vi "Sweep_AIWFM_time.vi"(8 "error in (no error)":errorcluster, 11 "Transport":refnum<class "Transport.lvclass">) -> (0 "error out":errorcluster, 3 "Transport.lvclass":refnum<class "Transport.lvclass">)   [LabVIEW 2019, in "Transport.lvclass"]
uses:
  Transport.lvclass
  <userlib>/LevyLab/Instrument Framework/Instrument Types/Cryostat/Instrument.Cryostat.lvclass
  Control Experiment/Control Experiment.lvclass
  Control Experiment/Typedefs/Instrument Classes--cluster.ctl
  <userlib>/LevyLab/Instrument Framework/Instrument Types/VSource/Instrument.VSource.lvclass
  <userlib>/LevyLab/Instrument Framework/Instrument Types/VNA/Instrument.VNA.lvclass
  <userlib>/LevyLab/Instrument Framework/Instrument Types/Strain/Instrument.Strain.lvclass
  <userlib>/LevyLab/Instrument Framework/Instrument Types/CBridge/Instrument.CBridge.lvclass
  <vilib>/Waveform/WDTOps.llb/WDT Append Waveforms DBL.vi
  <vilib>/PRIrvin/XY Utilities/xy_utilities.lvlib
  <vilib>/PRIrvin/XY Utilities/subVIs/Waveform to XY (single).vi
  <vilib>/PRIrvin/XY Utilities/subVIs/Get X and Y (single).vi
  <userlib>/LevyLab/Lockin-Multichannel/Instrument.DAQ/Typedefs/Sweep.Configuration--Cluster.ctl
  <userlib>/LevyLab/Lockin-Multichannel/Instrument.DAQ/Instrument.DAQ.lvclass
  <userlib>/LevyLab/Lockin-Multichannel/Instrument.DAQ/Typedefs/Sweep.Channel--Cluster.ctl
  <userlib>/LevyLab/Instrument Framework/Instrument Types/Delay Line/Instrument.DelayLine.lvclass
  <userlib>/LevyLab/Lockin-Multichannel/Instrument.DAQ/Typedefs/Sweep.Channel--Cluster--Array.ctl
  <userlib>/LevyLab/Instrument Framework/Instrument Types/Lockin/Instrument.LockinAPI.lvclass
  <userlib>/LevyLab/Instrument Framework/Instrument Types/Amplifier/Instrument.Amplifier.lvclass
  <userlib>/LevyLab/Lockin-Multichannel/Instrument.DAQ/Typedefs/Sweep.Pattern--Enum.ctl
  <userlib>/LevyLab/Lockin-Multichannel/Instrument.Lockin/Instrument.Lockin.lvclass
  <userlib>/LevyLab/Lockin-Multichannel/Instrument.DAQ/Typedefs/Get State-enum.ctl
panel:
  out "elapsed time (s)":u32=36594
  out "time b/w points (ms)":u32=533
  in  "Stop":bool
  in  "Tab Control":enum32{"Control", "Waveform", "Other"}(tab)
  in  "Sweep Time (s)":dbl=10.0 format="%#_3p"
  in  "Initial Wait (s)":u32=1
  in  "Return to Start":bool=TRUE
  in  "wait (ms)":u32=500
  in  "Experiment Description":string="SA40321H:\nT=80mK, BG=0V, B=-9T\nLoop 0: sgR: -1V to 1V, 20mV step\nInner loop: I+/I-: 28/2   -180mV to 220mV, sweep time 10s\nsgL (lead 1): 0V\nsgR (lead 3): sweep\n    \nI+/I-: 28/2   -180mV to 220mV, sweep time 10s\nV+/V-: 5/2\nsgL-lead 1; sgR-lead 3\n\ntc: 100ms\norder: 4\n\n"
  in  "Experiment Folder":string="01-sgR IV for RD"
  in  "Channels":T1[](array[typedef]) {"Table" format="%#_1f"; "Channel" min=1 max=128; "Start" format="%#_6p"; "End" format="%#_6p"}
  out "AO":waveform(dbl)(graph)={"t0"=timestamp(3666661573.979815 s since 1904-01-01), "dt"=0.0009999999996825864, "Y"=[]}
  out "AI vs AO":cluster{"Y":dbl[], "Y":dbl[]}[](graph)
  out "AI":waveform(dbl)[](graph)
  out "Status":T3=enum."created"
  out "Current State":string="File: Save"
  # "*** These controls are only read if this VI is the top level. If is is called from Sweep Control then the folder and comments come from Sweep Control.vi ***"
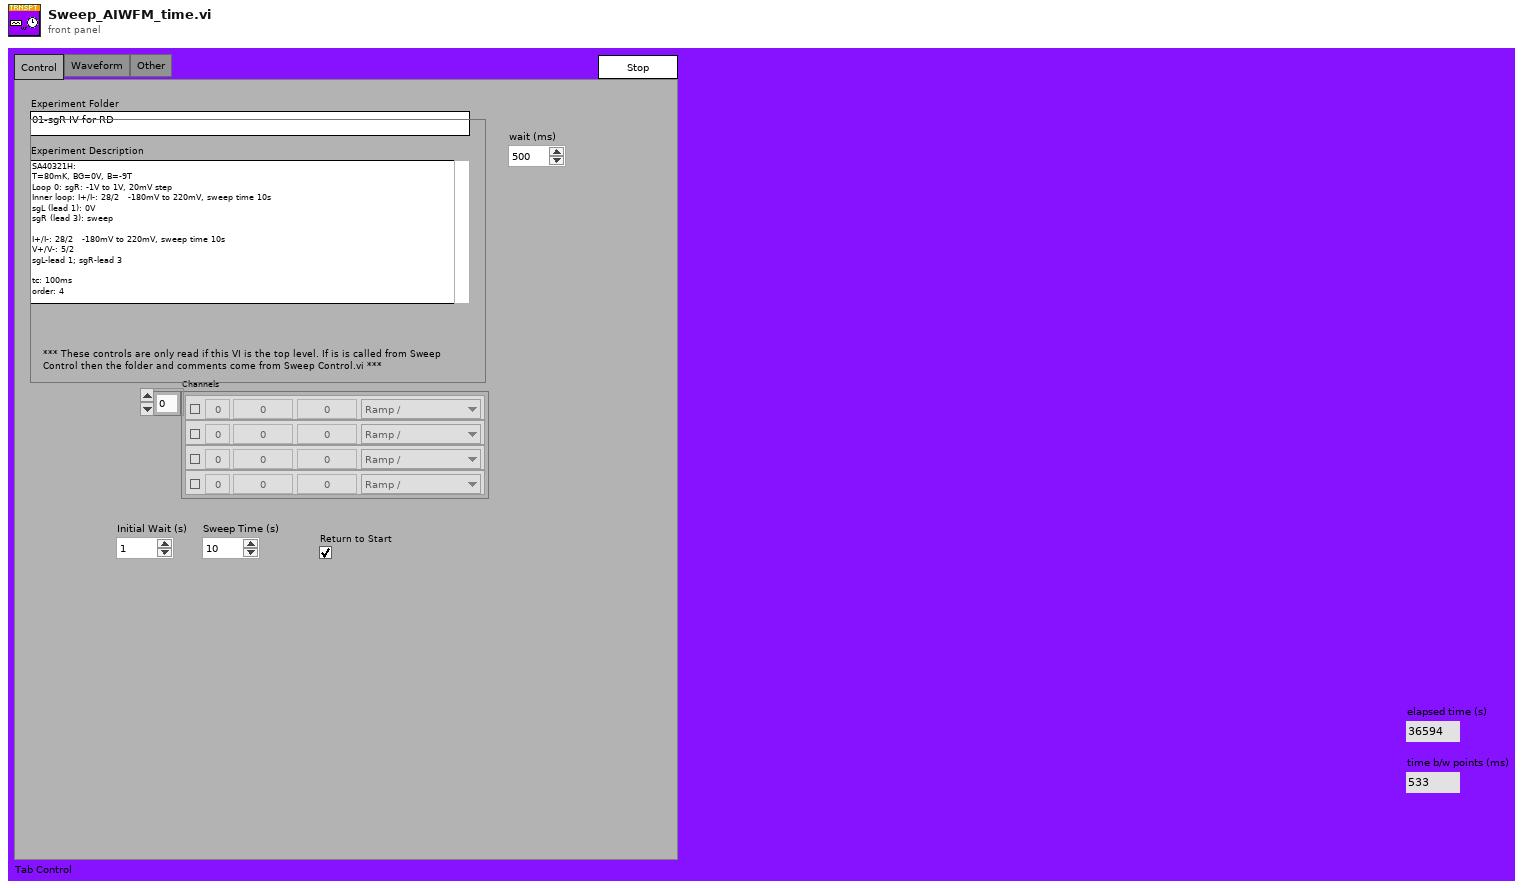
[diagram p1: front panel]
types:
  T1 = typedef "Instrument.Lockin.lvlib/Instrument.DAQ.lvclass/Sweep.Channel--Cluster.ctl" = cluster{"Enable?":bool, "Channel":u16, "Start":dbl, "End":dbl, "Pattern":T2, "Table":dbl[]}
  T2 = typedef "Instrument.Lockin.lvlib/Instrument.DAQ.lvclass/Sweep.Pattern--Enum.ctl" = enum16{"Ramp /", "Ramp /\\", "Smooth Ramp _/", "Smooth Ramp _/\\_", "Table"}
  T3 = typedef "Instrument.Lockin.lvlib/Instrument.DAQ.lvclass/Get State-enum.ctl" = enum16{"idle", "created", "started", "stopped", "sweeping"}
  T4 = enum32{"Invalid", "Standard", "Closed", "Hidden", "Minimized", "Maximized"}
  T5 = enum32{"invalid app kind", "Development System", "Run Time System", "Student Edition", "Embedded LabVIEW", "Evaluation", "Custom"}
  T6 = typedef "Control Experiment.lvclass/Instrument Classes--cluster.ctl" = cluster{"DAQ":refnum<class "Instrument.LockinAPI.lvclass">, "Amplifier":refnum<class "Instrument.Amplifier.lvclass">, "Temperature":refnum<class "Instrument.Cryostat.lvclass">, "Magnet":refnum<class "Instrument.Cryostat.lvclass">, "Rotator":refnum<class "Instrument.Cryostat.lvclass">, "Level":refnum<class "Instrument.Cryostat.lvclass">, "Capacitance":refnum<class "Instrument.CBridge.lvclass">, "Delay Line":refnum<class "Instrument.DelayLine.lvclass">, "Strain Cell":refnum<class "Instrument.Strain.lvclass">, "VNA":refnum<class "Instrument.VNA.lvclass">, "Source":refnum<class "Instrument.VSource.lvclass">}
  T7 = typedef "Instrument.Lockin.lvlib/Instrument.DAQ.lvclass/Sweep.Configuration--Cluster.ctl" = cluster{"Sweep Time (s)":dbl, "Initial Wait (s)":dbl, "Return to Start":bool, "Channels":T8}
  T8 = typedef "Instrument.Lockin.lvlib/Instrument.DAQ.lvclass/Sweep.Channel--Cluster--Array.ctl" = T1[]
  T9 = cluster{"Core":cluster{"Current VI Reference":refnum<vi>, "Close Panel on Exit?":bool}, "Transport":refnum<class "Transport.lvclass">, "C.E.":refnum<class "Control Experiment.lvclass">, "Notifier":refnum<notifier>, "Instruments":T6, "path":path, "time":dbl, "temperature":dbl, "magnet field":dbl, "AI XY (new)":cluster{dbl[], dbl[]}[], "AI XY (all)":cluster{dbl[], dbl[]}[], "AI Waveform (s)":waveform(dbl)[], "t0":timestamp, "ms [0]":u32, "ms [i]":u32, "AO Waveform (s)":waveform(dbl)[], "Execution:State":enum32{"Bad", "Idle", "Run top level", "Running"}}
  T10 = enum32{"Bad", "Idle", "Run top level", "Running"}
  T11 = cluster{"Current VI Reference":refnum<vi>, "Close Panel on Exit?":bool}
  T12 = typedef "Instrument.LockinAPI.lvclass/LockinAPI.getState.states--enum.ctl" = enum16{"idle", "created", "started", "stopped", "sweeping"}
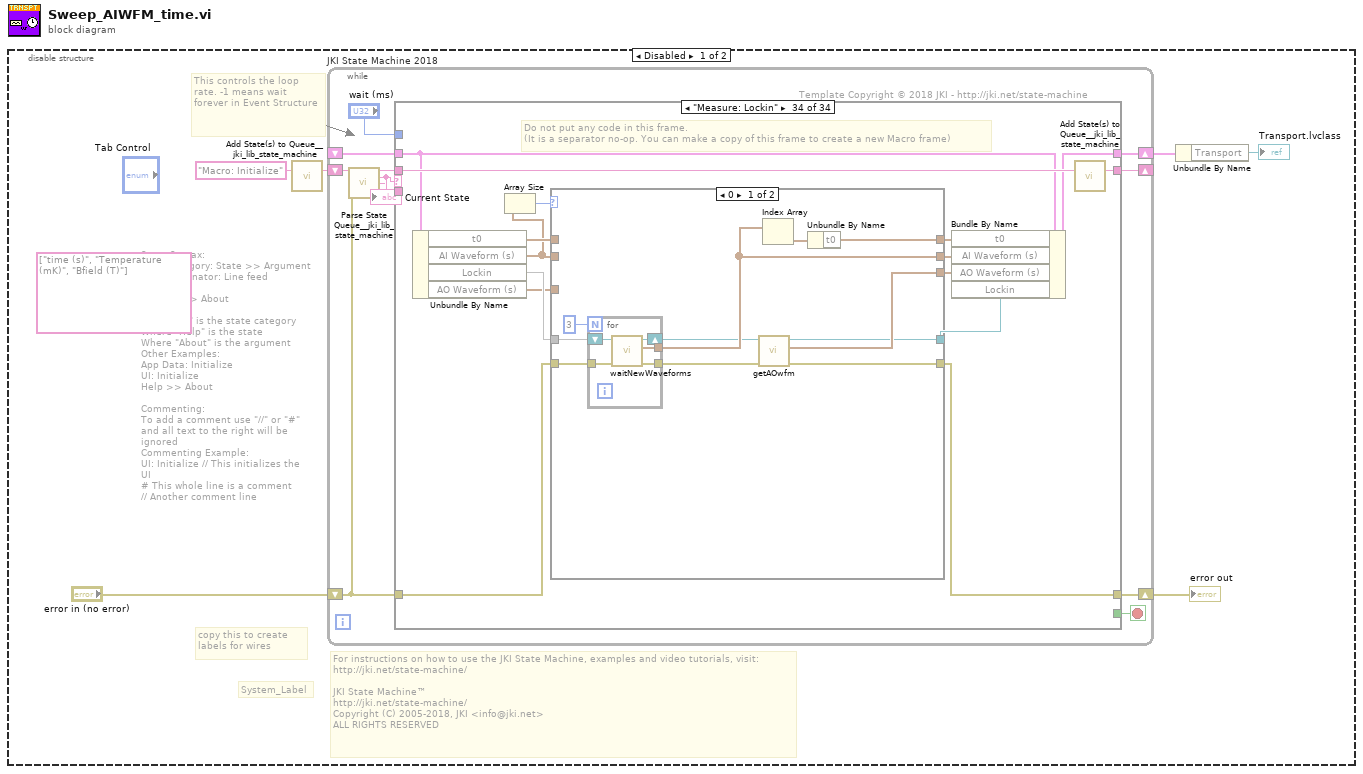
[diagram p0: block diagram]
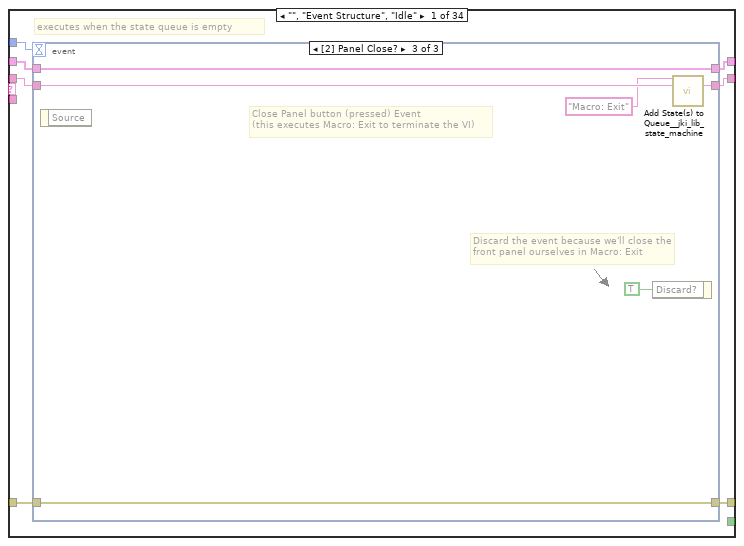
[diagram p2: hidden frame]
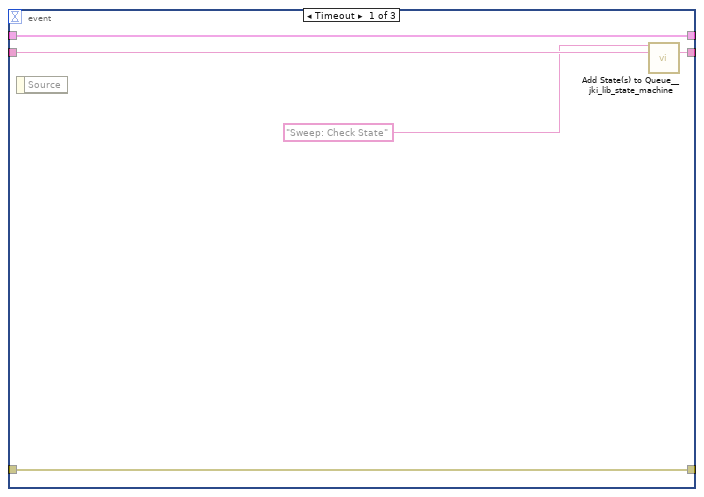
[diagram p3: hidden frame]
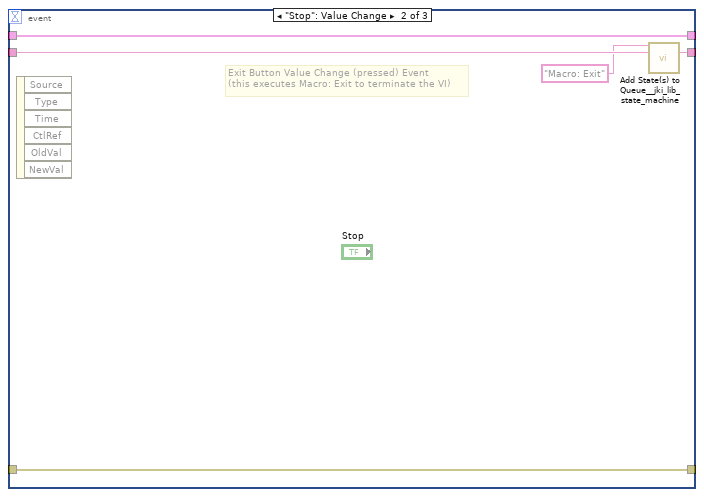
[diagram p4: hidden frame]
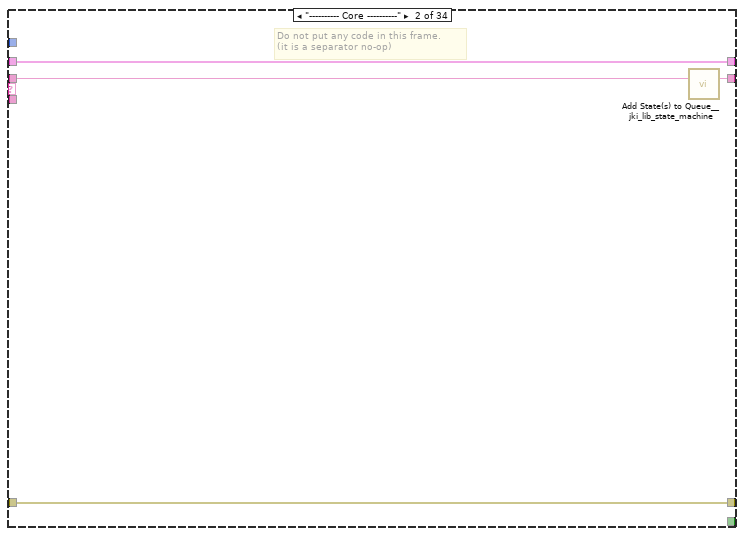
[diagram p5: hidden frame]
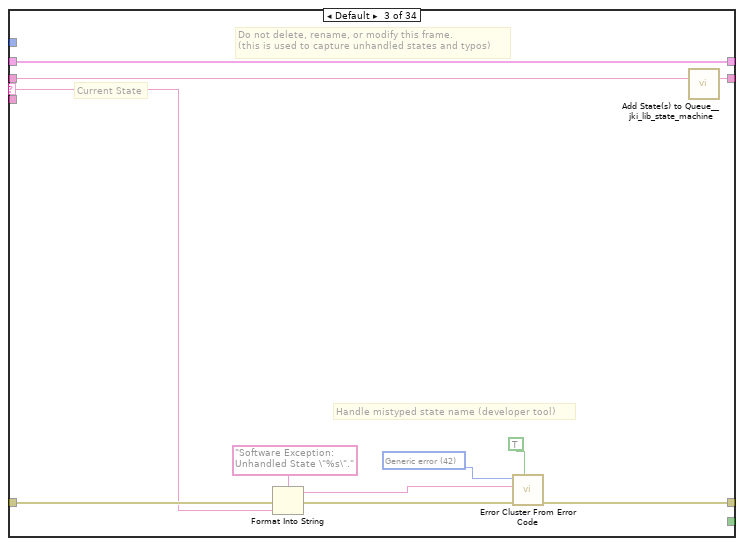
[diagram p6: hidden frame]
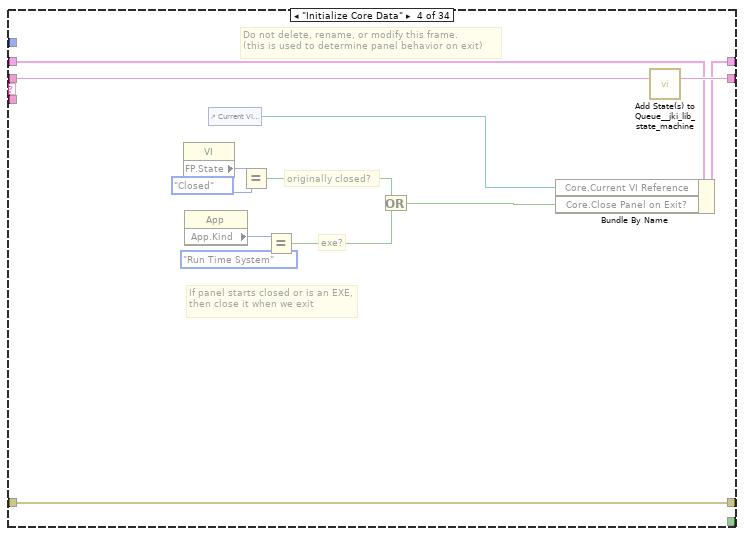
[diagram p7: hidden frame]
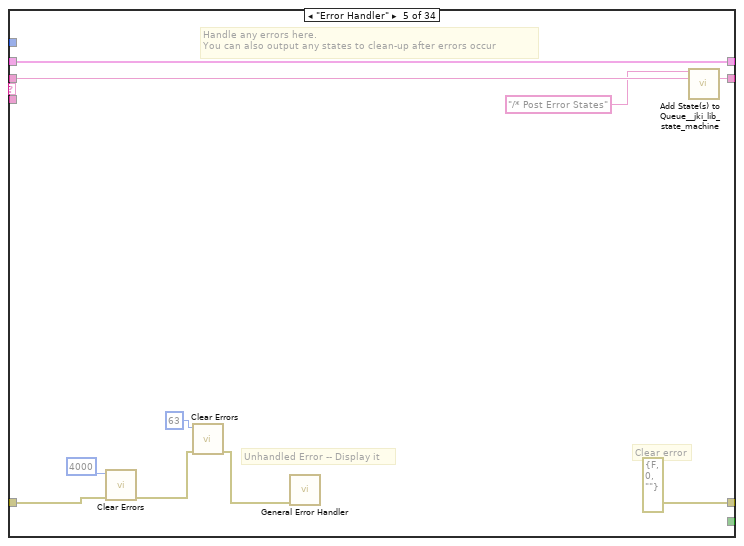
[diagram p8: hidden frame]
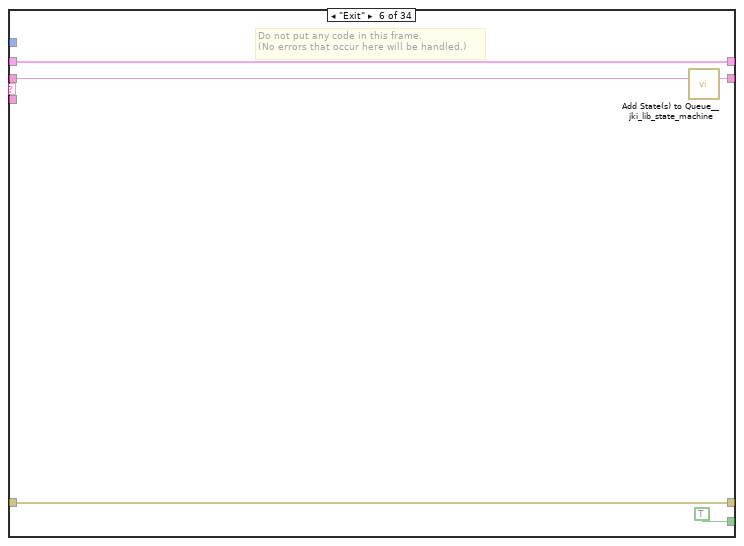
[diagram p9: hidden frame]
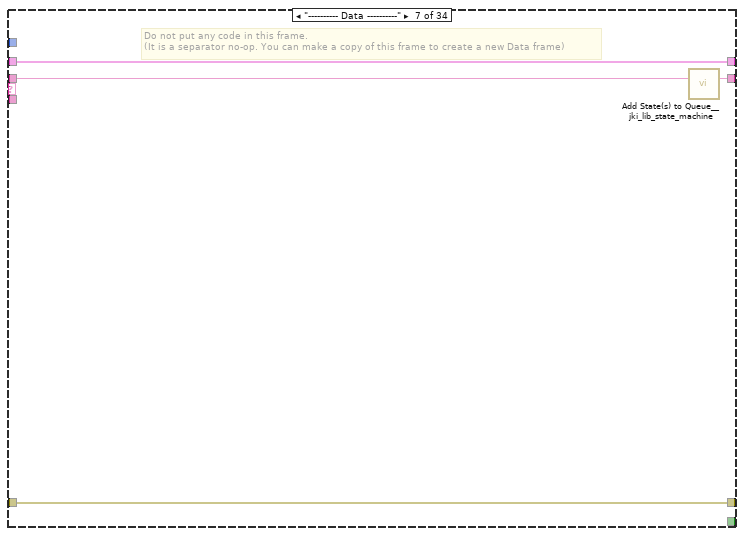
[diagram p10: hidden frame]
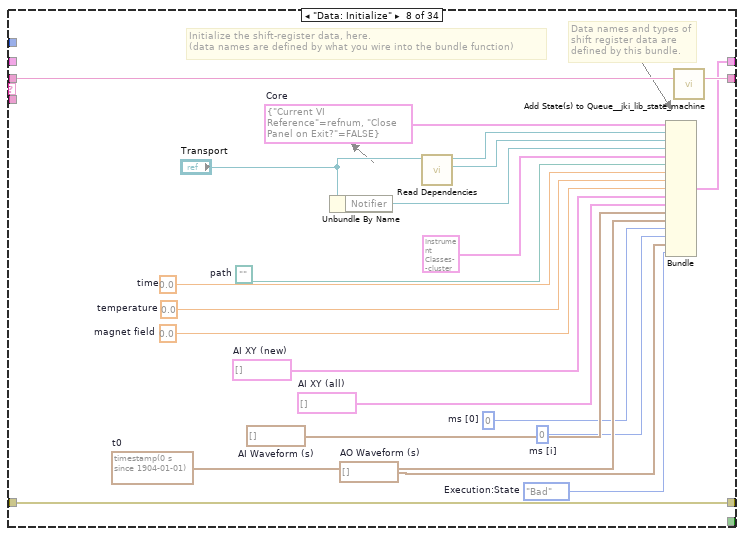
[diagram p11: hidden frame]
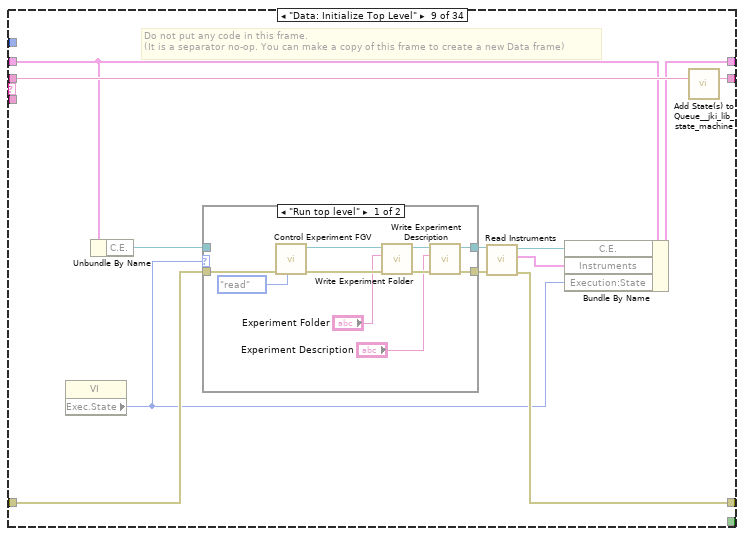
[diagram p12: hidden frame]
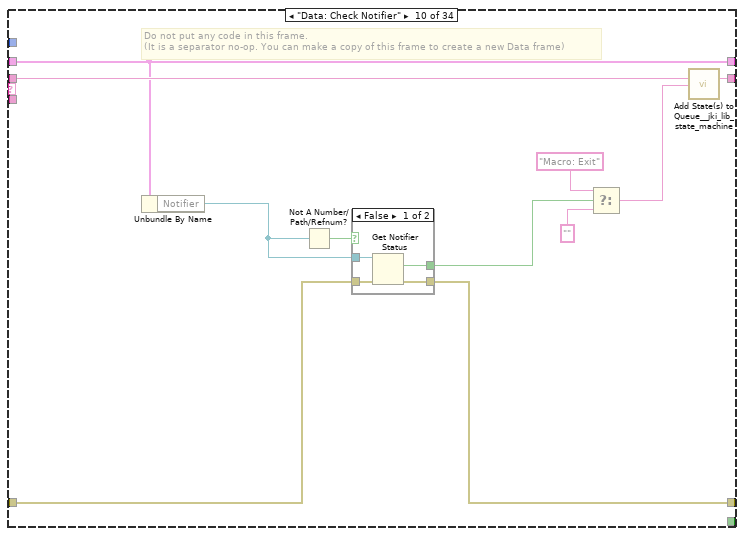
[diagram p14: hidden frame]
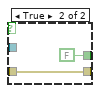
[diagram p15: hidden frame]
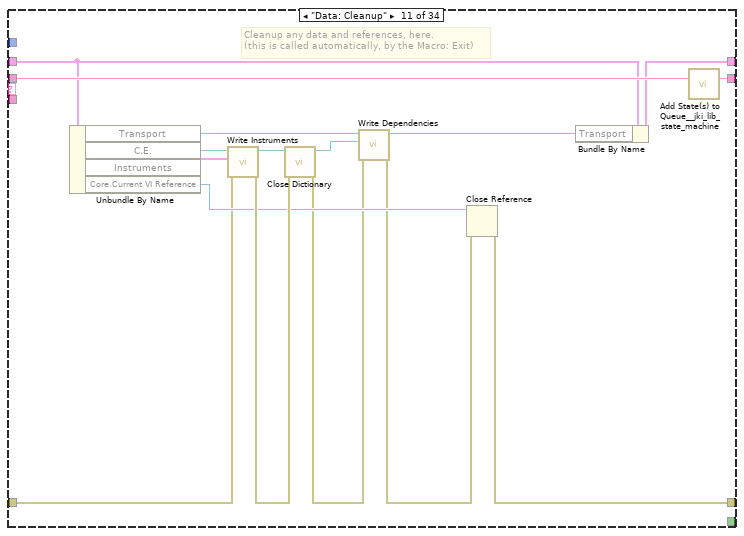
[diagram p16: hidden frame]
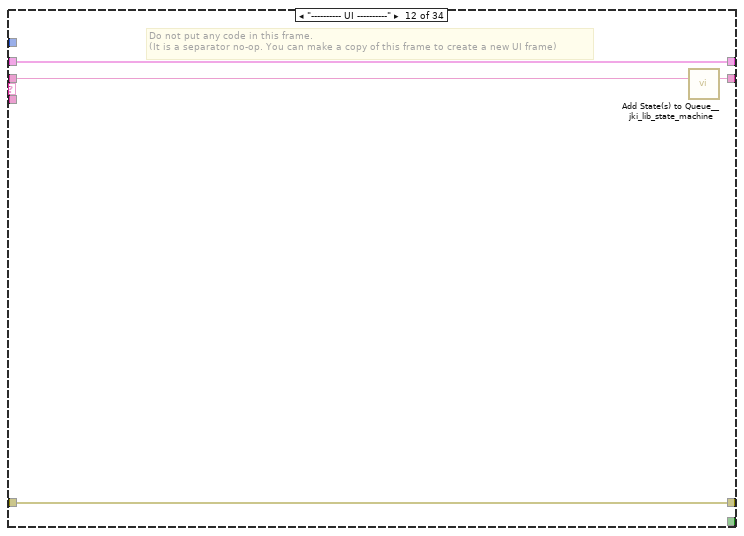
[diagram p17: hidden frame]
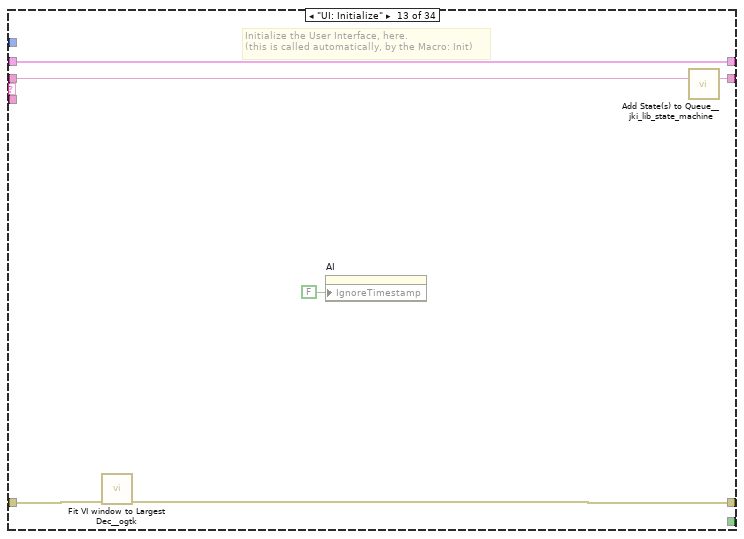
[diagram p18: hidden frame]
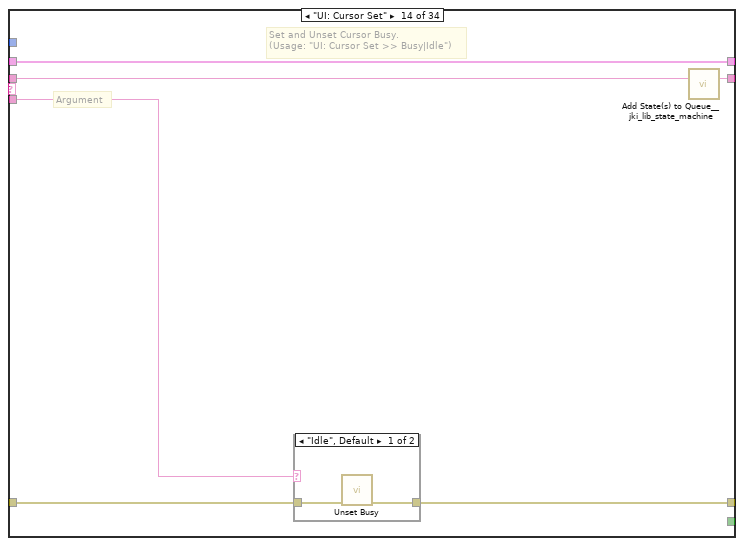
[diagram p19: hidden frame]
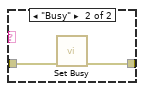
[diagram p20: hidden frame]
diagram:
  n1 = disable-structure shown="Disabled" {
    frame Disabled {
      (unwired) string[] ["time (s)", "Temperature (mK)", "Bfield (T)"] ("wavenames (.Vx, etc)")
      # "For instructions on how to use the JKI State Machine, examples and video tutorials, visit:\nhttp://jki.net/state-machine/\n\nJKI State Machine™\nhttp://jki.net/state-machine/\nCopyright (C) 2005-2018, JKI <info@jki.net>\nALL RIGHTS RESERVED"
      # "State Syntax:\nStateCategory: State >> Argument\nLine Terminator: Line feed\nExample:\nUI: Help >> About\n\nWhere \"UI\" is the state category\nWhere \"Help\" is the state\nWhere \"About\" is the argument\nOther Examples:\nApp Data: Initialize\nUI: Initialize\nHelp >> About\n\nCommenting:\nTo add a comment use \"//\" or \"#\" and all text to the right will be ignored\nCommenting Example:\nUI: Initialize // This initializes the UI\n# This whole line is a comment\n// Another comment line"
      # "copy this to create labels for wires"
      # "This controls the loop rate. -1 means wait forever in Event Structure"
      # "System_Label"
      n2 = call <vilib>:"Add State(s) to Queue__jki_lib_state_machine.vi"("State(s) in (\"\")"="Macro: Initialize") -> ("States Out"=w6:string)  [unwired: 14 in]
      n3 = while "JKI State Machine 2018" {
        shift-right: [w10] -> w2
        shift-left: _ -> [w9]
        shift-right: [w13] -> w3
        shift-left: "error in (no error)" -> [w8]
        shift-right: [w12] -> _
        shift-left: w6 -> [w14]
        stop <- w11 stop-if-true
        # "Template Copyright © 2018 JKI - http://jki.net/state-machine"
        n4 = call <vilib>:"Parse State Queue__jki_lib_state_machine.vi"("State Queue"=w14, "Error In (no error)"=w8) -> ("Remaining States"=w16:string, "Current State"=w17:string, "Arguments"=w15:string)  [unwired: 11 in]
        "Current State" <- w17
        n5 = case shown="\"Measure: Lockin\"" w17 {
          selector: w17 -> [_ _ w45 _ _ _ _ _ _ _ _ _ _ _ _ _ _ _ _ _ _ _ _ _ _ _ _ _ _ _ _ _ _ _]
          tunnel: w16 -> [w24 w44 w49 w68 w78 w83 w87 w109 w121 w144 w166 w170 w176 w182 w193 w270 w288 w292 w297 w302 w310 w320 w324 w347 w371 w387 w397 w405 w415 w421 w432 w445 w458 w473]
          tunnel: w15 -> [_ _ _ _ _ _ _ _ _ _ _ _ _ w177 w187 _ _ _ _ _ _ _ _ _ _ _ _ _ _ _ _ _ _ _]
          tunnel: w9 -> [w22 w41 w47 w61 w75 w81 w84 _ w117 w141 w153 w167 w174 w180 w189 w268 w276 w289 w294 w299 w307 w317 w321 w345 w368 w376 w390 w398 w406 w418 w428 w441 w456 w470]
          tunnel: [w21 w42 w51 w65 errorcluster {"status"=FALSE, "code"=0, "source"=""} ("error out") w80 w85 w106 w111 w140 w151 w168 w172 w178 w190 w267 w278 w290 w295 w300 w308 w318 w322 w344 w369 w384 w388 w401 w410 w419 w422 w434 w451 w464] -> w13
          tunnel: w8 -> [w20 w42 w50 w65 w72 w80 w85 w106 w116 w139 w152 w168 w173 w179 w191 w267 w279 w290 w295 w300 w308 w318 w322 w340 w369 w385 w394 w402 w411 w419 w425 w442 w450 w465]
          tunnel: [w23 w43 w48 w67 w77 w82 w86 w108 w120 w143 w165 w169 w175 w181 w192 w269 w287 w291 w296 w301 w309 w319 w323 w346 w370 w386 w396 w404 w414 w420 w431 w444 w457 w472] -> w12
          tunnel: [_ _ _ _ _ TRUE _ _ _ _ _ _ _ _ _ _ _ _ _ _ _ _ _ _ _ _ _ _ _ _ _ _ _ _] -> w11
          tunnel: [w19 w41 w47 w66 w75 w81 w84 w107 w118 w141 w154 w167 w174 w180 w189 w268 w277 w289 w294 w299 w307 w317 w321 w345 w368 w375 w391 w399 w407 w418 w429 w440 w455 w471] -> w10
          tunnel: "wait (ms)" -> [w18 _ _ _ _ _ _ _ _ _ _ _ _ _ _ _ _ _ _ _ _ _ _ _ _ _ _ _ _ _ _ _ _ _]
          frame "", "Event Structure", "Idle" {
            # "executes when the state queue is empty"
            n6 = event shown="[2] Panel Close?" {
              selector: _ -> [_ _ _]
              dyn-events: _ -> [_ _ _]
              timeout: w18 -> [_ _ _]
              tunnel: w24 -> [w29 w34 w40]
              tunnel: [w28 w33 w39] -> w23
              tunnel: w22 -> [w26 w31 w37]
              tunnel: [w27 w32 w38] -> w21
              tunnel: w20 -> [w27 w32 w38]
              tunnel: [w26 w31 w37] -> w19
              event Timeout {
                n7 = event-data() -> ()  [unwired: 1 in, 1 out]
                n8 = call <vilib>:"Add State(s) to Queue__jki_lib_state_machine.vi"("State(s) in Front (\"\")"="Sweep: Check State" ("State(s) in Front (\"\")"), "State(s) in (\"\")"=w29) -> ("States Out"=w28:string)  [unwired: 13 in]
              }
              event "Stop": Value Change {
                # "Exit Button Value Change (pressed) Event\n(this executes Macro: Exit to terminate the VI)"
                n9 = event-data() -> ()  [unwired: 1 in, 6 out]
                n10 = call <vilib>:"Add State(s) to Queue__jki_lib_state_machine.vi"("State(s) in Front (\"\")"="Macro: Exit", "State(s) in (\"\")"=w34) -> ("States Out"=w33:string)  [unwired: 13 in]
              }
              event Panel Close? {
                # "Discard the event because we'll close the front panel ourselves in Macro: Exit"
                # "Close Panel button (pressed) Event\n(this executes Macro: Exit to terminate the VI)"
                n11 = event-data() -> ()  [unwired: 1 in, 1 out]
                n12 = event-data("Discard?"=TRUE) -> ()  [unwired: 1 in, 1 out]
                n13 = call <vilib>:"Add State(s) to Queue__jki_lib_state_machine.vi"("State(s) in Front (\"\")"="Macro: Exit", "State(s) in (\"\")"=w40) -> ("States Out"=w39:string)  [unwired: 13 in]
              }
            }
          }
          frame "---------- Core ----------" {
            # "Do not put any code in this frame.\n(it is a separator no-op)"
            n14 = call <vilib>:"Add State(s) to Queue__jki_lib_state_machine.vi"("State(s) in (\"\")"=w44) -> ("States Out"=w43:string)  [unwired: 14 in]
          }
          frame Default {
            w54 = 42 items=["No error", "Argument error", "Memory is full", "Out of zone", "End of file", "File already open", "Generic file I/O error", "File not found", "File permission error", "Disk is full", "Duplicate path", "Too many files open", "System feature not enabled", "Resource file not found", "Cannot add resource", "Resource not found", "Image not found", "Image memory error", "Pen does not exist", "Config type invalid", "Config token not found", "Config parse error", "Config memory error", "Bad external code format", "Bad external code offset", "External code not present", "Null window", "Destroy window error", "Null menu", "Print aborted", "Bad print record", "Print driver error", "Windows error during printing", "Memory error during printing", "Print dialog error", "Generic print error", "Invalid device refnum", "Device not found", "Device parameter error", "Device unit error", "Cannot open device", "Device call aborted", "Generic error", "Cancelled by user", "Object ID too low", "Object ID too high", "Object not in heap", "Unknown heap", "Unknown object (invalid DefProc)", "Unknown object (DefProc not in table)", "Message out of range", "Invalid (null) method", "Unknown message", "Manager call not supported", "Bad address", "Network operation in progress", "Network operation timed out", "Connection is busy", "Network attribute not supported", "Network error", "Address in use", "System out of memory", "Connection aborted", "Connection refused", "Not connected", "Already connected", "Connection closed", "Initialization error (interapplication manager)", "Bad occurrence", "Wait on unbound occurrence handler", "Occurrence queue overflow", "Datalog type conflict", "Unused", "Unrecognized type (interapplication manager)", "Memory corrupt", "Failed to make temporary DLL", "Old CIN version", "Drag socket not found", "Failed to load drop-object", "Failed to register OLE object", "Failed to release OLE object", "Format specifier type mismatch", "Unknown format specifier", "Too few format specifiers", "Too many format specifiers", "Scan failed", "Newer CIN version", "Error converting to variant", "Runtime menu error", "Password tampered", "Variant attribute not found", "Incompatible variant data type", "Event data is not available", "Event Store is not present", "Occurrence is not found", "Event Queue is not created", "Event info is not available", "Refnum passed is NULL", "Error retrieving Class GUID", "Error retrieving CoClass GUID", "Error retrieving TypeLib GUID.", "Bad built application magic bytes.", "Specific driver is different from the specific driver associated with the Logical Name.", "There is no session opened to the class driver.", "Max Error", "MAX - Error with config objects", "MAX - Error loading configuration", "MAX - Group not supported"]
            # "Current State"
            # "Do not delete, rename, or modify this frame.\n(this is used to capture unhandled states and typos)"
            # "Handle mistyped state name (developer tool)"
            n15 = Format Into String(format string="Software Exception: Unhandled State \"%s\"." ("message"), error in=w50, w45) -> (resulting string=w53:string, error out=w52:errorcluster)  [unwired: 1 in]
            n16 = call <vilib>:"Error Cluster From Error Code.vi"("show call chain? (False)"=TRUE, "error in (no error)"=w52, "error message (\"\")"=w53, "error code (0)"=w54) -> ("error out"=w51:errorcluster)  [unwired: 5 in]
            n17 = call <vilib>:"Add State(s) to Queue__jki_lib_state_machine.vi"("State(s) in (\"\")"=w49) -> ("States Out"=w48:string)  [unwired: 14 in]
          }
          frame "Initialize Core Data" {
            # "Do not delete, rename, or modify this frame.\n(this is used to determine panel behavior on exit)"
            # "originally closed?"
            # "exe?"
            # "If panel starts closed or is an EXE, then close it when we exit"
            n18 = property class="VI"() -> ("FP.State"=w58:T4)  [unwired: 2 in, 2 out]
            n19 = property class="App"() -> ("App.Kind"=w64:T5)  [unwired: 2 in, 2 out]
            n20 = control-ref of="Current VI Reference"() -> (w59:refnum<vi>)
            n21 = Equal?(x=w58, y=T4."Closed" ("Front Panel Window:State")) -> (x = y?=w56:bool)
            n22 = Equal?(x=w64, y=T5."Run Time System" ("Application:Kind")) -> (x = y?=w62:bool)
            n23 = Or(x=w56, y=w62) -> (x .or. y?=w60:bool)
            n24 = Bundle By Name(cluster=w61, "Core.Current VI Reference"=w59, "Core.Close Panel on Exit?"=w60) -> (w66:T9)
            n25 = call <vilib>:"Add State(s) to Queue__jki_lib_state_machine.vi"("State(s) in (\"\")"=w68) -> ("States Out"=w67:string)  [unwired: 14 in]
          }
          frame "Error Handler" {
            # "Unhandled Error -- Display it"
            # "Handle any errors here.\nYou can also output any states to clean-up after errors occur"
            # "Clear error"
            n26 = call <vilib>:"Clear Errors.vi"("error in (no error)"=w72, "specific error code to clear (0: all)"=4000) -> ("error out"=w70:errorcluster)  [unwired: 4 in, 1 out]
            n27 = call <vilib>:"Clear Errors.vi"("error in (no error)"=w70, "specific error code to clear (0: all)"=63) -> ("error out"=w69:errorcluster)  [unwired: 4 in, 1 out]
            n28 = call <vilib>:"General Error Handler.vi"("error in (no error)"=w69) -> ()  [unwired: 10 in, 5 out]
            n29 = call <vilib>:"Add State(s) to Queue__jki_lib_state_machine.vi"("State(s) in Front (\"\")"="/* Post Error States", "State(s) in (\"\")"=w78) -> ("States Out"=w77:string)  [unwired: 13 in]
          }
          frame "Exit" {
            # "Do not put any code in this frame.\n(No errors that occur here will be handled.)"
            n30 = call <vilib>:"Add State(s) to Queue__jki_lib_state_machine.vi"("State(s) in (\"\")"=w83) -> ("States Out"=w82:string)  [unwired: 14 in]
          }
          frame "---------- Data ----------" {
            # "Do not put any code in this frame.\n(It is a separator no-op. You can make a copy of this frame to create a new Data frame)"
            n31 = call <vilib>:"Add State(s) to Queue__jki_lib_state_machine.vi"("State(s) in (\"\")"=w87) -> ("States Out"=w86:string)  [unwired: 14 in]
          }
          frame "Data: Initialize" {
            w93 = T10."Bad"  # Execution:State
            w94 = waveform(dbl)[] []  # AO Waveform (s)
            w89 = u32 0  # ms [i]
            w88 = u32 0  # ms [0]
            w95 = timestamp(0 s since 1904-01-01)  # t0
            w96 = waveform(dbl)[] []  # AI Waveform (s)
            w101 = cluster{dbl[], dbl[]}[] []  # AI XY (new)
            w102 = cluster{dbl[], dbl[]}[] []  # AI XY (all)
            w99 = 0.0  # magnet field
            w98 = 0.0  # temperature
            w97 = 0.0  # time
            w104 = path ""  # path
            w105 = T11 {"Current VI Reference"=refnum, "Close Panel on Exit?"=FALSE}  # Core
            # "Data names and types of shift register data are defined by this bundle."
            # "Initialize the shift-register data, here.\n(data names are defined by what you wire into the bundle function)"
            n32 = Unbundle By Name("Transport") -> ("Notifier"=w103:refnum<notifier>)
            n33 = call "Read Dependencies.vi"("Transport"="Transport") -> ("C.E."=w91:refnum<class "Control Experiment.lvclass">, "Transport"=w90:refnum<class "Transport.lvclass">)  [unwired: 8 in, 1 out]
            n34 = Bundle("Core"=w105, "Transport"=w90, "C.E."=w91, "Notifier"=w103, "Instruments"=T6 {"DAQ"=refnum, "Amplifier"=refnum, "Temperature"=refnum, "Magnet"=refnum, "Rotator"=refnum, "Level"=refnum, "Capacitance"=refnum, "Delay Line"=refnum, "Strain Cell"=refnum, "VNA"=refnum, "Source"=refnum}, "path"=w104, "time"=w97, "temperature"=w98, "magnet field"=w99, "AI XY (new)"=w101, "AI XY (all)"=w102, "AI Waveform (s)"=w96, "t0"=w95, "ms [0]"=w88, "ms [i]"=w89, "AO Waveform (s)"=w94, "Execution:State"=w93) -> (w107:T9)  [unwired: 1 in]
            n35 = call <vilib>:"Add State(s) to Queue__jki_lib_state_machine.vi"("State(s) in (\"\")"=w109) -> ("States Out"=w108:string)  [unwired: 14 in]
          }
          frame "Data: Initialize Top Level" {
            # "Do not put any code in this frame.\n(It is a separator no-op. You can make a copy of this frame to create a new Data frame)"
            n36 = property class="VI"() -> ("Exec.State"=w110:T10)  [unwired: 2 in, 2 out]
            n37 = Unbundle By Name(w117) -> ("C.E."=w119:refnum<class "Control Experiment.lvclass">)
            n38 = case shown="\"Run top level\"" w110 {
              tunnel: w116 -> [w131 w132]
              tunnel: [w126 w132] -> w115
              tunnel: [w125 w133] -> w114
              tunnel: w119 -> [_ w133]
              frame "Run top level" {
                n39 = call "Control Experiment FGV.vi"("Function"=enum16{"read", "write"}."read", "error in (no error)"=w131) -> ("error out"=w129:errorcluster, "Control Experiment.lvclass out"=w130:refnum<class "Control Experiment.lvclass">)  [unwired: 8 in]
                n40 = call "Write Experiment Folder.vi"("error in (no error)"=w129, "Experiment Folder"="Experiment Folder", "Control Experiment in"=w130) -> ("error out"=w127:errorcluster, "Control Experiment out"=w128:refnum<class "Control Experiment.lvclass">)  [unwired: 7 in]
                n41 = call "Write Experiment Description.vi"("error in (no error)"=w127, "Experiment Description"="Experiment Description", "Control Experiment in"=w128) -> ("error out"=w126:errorcluster, "Control Experiment out"=w125:refnum<class "Control Experiment.lvclass">)  [unwired: 7 in]
              }
              frame "Running", Default {
              }
            }
            n42 = call "Read Instruments.vi"("error in (no error)"=w115, "Control Experiment in"=w114) -> ("error out"=w111:errorcluster, "Instruments"=w112:T6, "Control Experiment out"=w113:refnum<class "Control Experiment.lvclass">)  [unwired: 7 in]
            n43 = Bundle By Name(cluster=w117, "C.E."=w113, "Instruments"=w112, "Execution:State"=w110) -> (w118:T9)
            n44 = call <vilib>:"Add State(s) to Queue__jki_lib_state_machine.vi"("State(s) in (\"\")"=w121) -> ("States Out"=w120:string)  [unwired: 14 in]
          }
          frame "Data: Check Notifier" {
            # "Do not put any code in this frame.\n(It is a separator no-op. You can make a copy of this frame to create a new Data frame)"
            n45 = Unbundle By Name(w141) -> ("Notifier"=w134:refnum<notifier>)
            n46 = Not A Number/Path/Refnum?(number/path/refnum=w134) -> (NaN/Path/Refnum?=w142:bool)
            n47 = case shown="False" w142 {
              tunnel: [w148 FALSE] -> w138
              tunnel: [w147 w149] -> w140
              tunnel: w134 -> [w146 _]
              tunnel: w139 -> [w145 w149]
              frame False {
                n48 = Get Notifier Status(notifier=w146, error in (no error)=w145) -> (current notification=w148:bool, error out=w147:errorcluster)  [unwired: 3 out]
              }
              frame True {
              }
            }
            n49 = Select(t="Macro: Exit", s=w138, f="") -> (s? t:f=w135:string)
            n50 = call <vilib>:"Add State(s) to Queue__jki_lib_state_machine.vi"("State(s) in (\"\")"=w144, "State(s) at Back (\"\")"=w135) -> ("States Out"=w143:string)  [unwired: 13 in]
          }
          frame "Data: Cleanup" {
            # "Cleanup any data and references, here.\n(this is called automatically, by the Macro: Exit)"
            n51 = Unbundle By Name(w153) -> ("Transport"=w162:refnum<class "Transport.lvclass">, "C.E."=w164:refnum<class "Control Experiment.lvclass">, "Instruments"=w159:T6, "Core.Current VI Reference"=w157:refnum<vi>)
            n52 = call "Write Instruments.vi"("error in (no error)"=w152, "Instruments"=w159, "Control Experiment in"=w164) -> ("error out"=w158:errorcluster, "Control Experiment out"=w160:refnum<class "Control Experiment.lvclass">)  [unwired: 7 in]
            n53 = call "Close Dictionary.vi"("error in (no error)"=w158, "Control Experiment in"=w160) -> ("error out"=w156:errorcluster, "Control Experiment out"=w161:refnum<class "Control Experiment.lvclass">)  [unwired: 8 in]
            n54 = call "Write Dependencies.vi"("error in (no error)"=w156, "Control Experiment"=w161, "Transport in"=w162) -> ("error out"=w155:errorcluster, "Transport out"=w163:refnum<class "Transport.lvclass">)  [unwired: 7 in]
            n55 = Close Reference(reference=w157, error in (no error)=w155) -> (error out=w151:errorcluster)
            n56 = Bundle By Name(cluster=w153, "Transport"=w163) -> (w154:T9)
            n57 = call <vilib>:"Add State(s) to Queue__jki_lib_state_machine.vi"("State(s) in (\"\")"=w166) -> ("States Out"=w165:string)  [unwired: 14 in]
          }
          frame "---------- UI ----------" {
            # "Do not put any code in this frame.\n(It is a separator no-op. You can make a copy of this frame to create a new UI frame)"
            n58 = call <vilib>:"Add State(s) to Queue__jki_lib_state_machine.vi"("State(s) in (\"\")"=w170) -> ("States Out"=w169:string)  [unwired: 14 in]
          }
          frame "UI: Initialize" {
            # "Initialize the User Interface, here.\n(this is called automatically, by the Macro: Init)"
            n59 = call <userlib>:"Fit VI window to Largest Dec__ogtk.vi"("error in (no error)"=w173) -> ("error out"=w172:errorcluster)  [unwired: 5 in, 1 out]
            n60 = property on="AI" class="WFGraph (strict)"("IgnoreTimestamp"=FALSE ("Ignore Timestamp")) -> ()  [unwired: 2 in, 2 out]
            n61 = call <vilib>:"Add State(s) to Queue__jki_lib_state_machine.vi"("State(s) in (\"\")"=w176) -> ("States Out"=w175:string)  [unwired: 14 in]
          }
          frame "UI: Cursor Set" {
            # "Argument"
            # "Set and Unset Cursor Busy.\n(Usage: \"UI: Cursor Set >> Busy|Idle\")"
            n62 = case shown="\"Idle\", Default" w177 {
              tunnel: w179 -> [w184 w186]
              tunnel: [w183 w185] -> w178
              frame "Idle", Default {
                n63 = call <vilib>:"Unset Busy.vi"("error in (no error)"=w184) -> ("error out"=w183:errorcluster)  [unwired: 10 in]
              }
              frame "Busy" {
                n64 = call <vilib>:"Set Busy.vi"("error in (no error)"=w186) -> ("error out"=w185:errorcluster)  [unwired: 9 in, 1 out]
              }
            }
            n65 = call <vilib>:"Add State(s) to Queue__jki_lib_state_machine.vi"("State(s) in (\"\")"=w182) -> ("States Out"=w181:string)  [unwired: 14 in]
          }
          frame "UI: Front Panel State" {
            # "Argument"
            # "Set Front Panel Open or Closed\n(Usage: \"UI: Front Panel State >> Open|Close\")"
            n66 = Unbundle By Name(w189) -> ("Core.Current VI Reference"=w188:refnum<vi>)
            n67 = case shown="\"Minimize\", \"Minimized\"" w187 {
              tunnel: w191 -> [w199 w214 w225 w238 w251]
              tunnel: [w201 w215 w227 w240 w253] -> w190
              tunnel: w188 -> [w200 w212 w226 w239 w252]
              frame "Open", "Standard", Default {
                w194 = T4."Standard" ("State")
                n68 = property class="VI"(reference=w200, error in=w199) -> (reference out=w197:refnum<vi>, error out=w198:errorcluster, "FP.State"=w196:T4)
                n69 = Not Equal?(x=w196, y=w194) -> (x != y?=w195:bool)
                n70 = case shown="True" w195 {
                  tunnel: [w205 w207] -> w201
                  tunnel: w198 -> [w204 w207]
                  tunnel: w197 -> [w203 _]
                  tunnel: w194 -> [w202 _]
                  frame True {
                    n71 = invoke class="VI" method="FP.Open"(reference=w203, error in=w204, "Activate"=TRUE, "State"=w202) -> (error out=w205:errorcluster)  [unwired: 1 in, 4 out]
                  }
                  frame False {
                  }
                }
              }
              frame "Close", "Closed" {
                n72 = property class="VI"(reference=w212, error in=w214) -> (reference out=w211:refnum<vi>, error out=w213:errorcluster, "FP.State"=w209:T4)
                n73 = Not Equal?(x=w209, y=T4."Closed" ("Front Panel Window:State")) -> (x != y?=w208:bool)
                n74 = case shown="True" w208 {
                  tunnel: [w216 w219] -> w215
                  tunnel: w213 -> [w216 w218]
                  tunnel: w211 -> [_ w217]
                  frame False {
                  }
                  frame True {
                    n75 = invoke class="VI" method="FP.Close"(reference=w217, error in=w218) -> (error out=w219:errorcluster)  [unwired: 1 in, 2 out]
                  }
                }
              }
              frame "Hidden", "Hide" {
                w220 = T4."Hidden" ("State")
                n76 = property class="VI"(reference=w226, error in=w225) -> (reference out=w223:refnum<vi>, error out=w224:errorcluster, "FP.State"=w222:T4)
                n77 = Not Equal?(x=w222, y=w220) -> (x != y?=w221:bool)
                n78 = case shown="True" w221 {
                  tunnel: [w231 w232] -> w227
                  tunnel: w224 -> [w230 w232]
                  tunnel: w223 -> [w229 _]
                  tunnel: w220 -> [w228 _]
                  frame True {
                    n79 = invoke class="VI" method="FP.Open"(reference=w229, error in=w230, "State"=w228) -> (error out=w231:errorcluster)  [unwired: 2 in, 4 out]
                  }
                  frame False {
                  }
                }
              }
              frame "Minimize", "Minimized" {
                w233 = T4."Minimized" ("State")
                n80 = property class="VI"(reference=w239, error in=w238) -> (reference out=w236:refnum<vi>, error out=w237:errorcluster, "FP.State"=w235:T4)
                n81 = Not Equal?(x=w235, y=w233) -> (x != y?=w234:bool)
                n82 = case shown="True" w234 {
                  tunnel: [w244 w245] -> w240
                  tunnel: w237 -> [w243 w245]
                  tunnel: w236 -> [w242 _]
                  tunnel: w233 -> [w241 _]
                  frame True {
                    n83 = invoke class="VI" method="FP.Open"(reference=w242, error in=w243, "State"=w241) -> (error out=w244:errorcluster)  [unwired: 2 in, 4 out]
                  }
                  frame False {
                  }
                }
              }
              frame "Maximize", "Maximized" {
                w246 = T4."Maximized" ("State")
                n84 = property class="VI"(reference=w252, error in=w251) -> (reference out=w249:refnum<vi>, error out=w250:errorcluster, "FP.State"=w248:T4)
                n85 = Not Equal?(x=w248, y=w246) -> (x != y?=w247:bool)
                n86 = case shown="True" w247 {
                  tunnel: [w257 w258] -> w253
                  tunnel: w250 -> [w256 w258]
                  tunnel: w249 -> [w255 _]
                  tunnel: w246 -> [w254 _]
                  frame True {
                    n87 = invoke class="VI" method="FP.Open"(reference=w255, error in=w256, "State"=w254) -> (error out=w257:errorcluster)  [unwired: 2 in, 4 out]
                  }
                  frame False {
                  }
                }
              }
            }
            n88 = call <vilib>:"Add State(s) to Queue__jki_lib_state_machine.vi"("State(s) in (\"\")"=w193) -> ("States Out"=w192:string)  [unwired: 14 in]
          }
          frame "UI: Update Graphs" {
            # "Do not put any code in this frame.\n(It is a separator no-op. You can make a copy of this frame to create a new UI frame)"
            n89 = local read "Channels"() -> (w264:T1[])
            n90 = Index Array(array=w264) -> (element=w263:T1)  [unwired: 1 in]
            n91 = Unbundle By Name(w268) -> ("AI Waveform (s)"=w266:waveform(dbl)[], "AO Waveform (s)"=w265:waveform(dbl)[])
            "AI" <- w266
            n92 = Unbundle By Name(w263) -> ("Channel"=w259:u16)
            n93 = Decrement(x=w259) -> (x-1=w262:u16)
            n94 = Index Array(array=w265, index=w262) -> (element=w260:waveform(dbl))
            "AO" <- w260
            n95 = for {
              tunnel: w266 -> [w275] mode=indexing
              tunnel: w260 -> [w274]
              tunnel: [w271] -> w261 mode=indexing
              n96 = Unbundle By Name(w274) -> ("Y"=w272:dbl[])
              n97 = Unbundle By Name(w275) -> ("Y"=w273:dbl[])
              n98 = Bundle("Y"=w272, "Y"=w273) -> (w271:cluster{"Y":dbl[], "Y":dbl[]})  [unwired: 1 in]
            }
            "AI vs AO" <- w261
            n99 = call <vilib>:"Add State(s) to Queue__jki_lib_state_machine.vi"("State(s) in (\"\")"=w270) -> ("States Out"=w269:string)  [unwired: 14 in]
          }
          frame "UI: Update Timer" {
            # "Do not put any code in this frame.\n(It is a separator no-op. You can make a copy of this frame to create a new UI frame)"
            n100 = Unbundle By Name(w276) -> ("ms [0]"=w281:u32)
            n101 = call <userlib>:"Tick Count (ms)__ogtk.vi"("error in (no error)"=w279) -> ("error out"=w285:errorcluster, "millisecond timer value"=w286:u32)  [unwired: 9 in]
            n102 = Subtract(x=w286, y=w281) -> (x-y=w283:u32)
            n103 = call <userlib>:"MGI Milliseconds Since Last Call.vi"("Error In"=w285) -> ("ms"=→"time b/w points (ms)":u32, "Error Out"=w278:errorcluster)  [unwired: 5 in]
            n104 = Divide(x=w283, y=u32 1000 ("x")) -> (x/y=→"elapsed time (s)":dbl)
            n105 = Bundle By Name(cluster=w276, "ms [i]"=w286) -> (w277:T9)
            n106 = call <vilib>:"Add State(s) to Queue__jki_lib_state_machine.vi"("State(s) in (\"\")"=w288) -> ("States Out"=w287:string)  [unwired: 14 in]
          }
          frame "---------- Macro ----------" {
            # "Do not put any code in this frame.\n(It is a separator no-op. You can make a copy of this frame to create a new Macro frame)"
            n107 = call <vilib>:"Add State(s) to Queue__jki_lib_state_machine.vi"("State(s) in (\"\")"=w292) -> ("States Out"=w291:string)  [unwired: 14 in]
          }
          frame "Macro: Initialize" {
            w293 = "Data: Initialize\nInitialize Core Data\nUI: Initialize\nUI: Front Panel State >> Open\nData: Initialize Top Level\nSweep: Initialize\nSweep: Start"  # Data: Initialize Initialize Core Data UI: Initialize UI: Front Panel State >> Open Data: Initialize Top Level Sweep: Initialize Sweep: Start
            # "Initialization Macro\n(This is called once, when the VI starts)"
            n108 = call <vilib>:"Add State(s) to Queue__jki_lib_state_machine.vi"("State(s) in Front (\"\")"=w293, "State(s) in (\"\")"=w297) -> ("States Out"=w296:string)  [unwired: 13 in]
          }
          frame "Macro: Sweep" {
            # "Initialization Macro\n(This is called once, when the VI starts)"
            n109 = call <vilib>:"Add State(s) to Queue__jki_lib_state_machine.vi"("State(s) in Front (\"\")"="Measure: Time\nMeasure: Lockin\nUI: Update Graphs\nUI: Update Timer", "State(s) in (\"\")"=w302) -> ("States Out"=w301:string)  [unwired: 13 in]
          }
          frame "Macro: Measure" {
            # "Initialization Macro\n(This is called once, when the VI starts)"
            n110 = call <vilib>:"Add State(s) to Queue__jki_lib_state_machine.vi"("State(s) in Front (\"\")"="Measure: Time\n//Measure: Temperature\n//Measure: Magnet\nMeasure: Lockin\nUI: Update Graphs", "State(s) in (\"\")"="", "State(s) at Back (\"\")"="Data: Check Notifier") -> ("States Out"=w305:string)  [unwired: 12 in]
            n111 = call <vilib>:"Add State(s) to Queue__jki_lib_state_machine.vi"("State(s) in Front (\"\")"=w305, "State(s) in (\"\")"=w310) -> ("States Out"=w309:string)  [unwired: 13 in]
          }
          frame "Macro: Exit" {
            # "Exit Macro\n(This is called once, when the VI exits)"
            n112 = Unbundle By Name(w317) -> ("Core.Close Panel on Exit?"=w316:bool)
            n113 = Select(t="UI: Front Panel State >> Close", s=w316, f="") -> (s? t:f=w313:string)
            n114 = call <vilib>:"Add State(s) to Queue__jki_lib_state_machine.vi"("State(s) in (\"\")"=w313, "State(s) at Back (\"\")"="Sweep: Stop\nFile: Save\nData: Cleanup\nExit") -> ("States Out"=w311:string)  [unwired: 13 in]
            n115 = call <vilib>:"Add State(s) to Queue__jki_lib_state_machine.vi"("State(s) in Front (\"\")"=w311, "State(s) in (\"\")"=w320) -> ("States Out"=w319:string)  [unwired: 13 in]
          }
          frame "---------- File ----------" {
            # "Template Separator\n(You can make a copy of, or modify, this frame)"
            n116 = call <vilib>:"Add State(s) to Queue__jki_lib_state_machine.vi"("State(s) in (\"\")"=w324) -> ("States Out"=w323:string)  [unwired: 14 in]
          }
          frame "File: Save" {
            # "Your code here.\n(You can make a copy of, or modify, this frame)"
            n117 = Unbundle By Name(w345) -> ("Execution:State"=w327:T10, "C.E."=w341:refnum<class "Control Experiment.lvclass">, "AI Waveform (s)"=w342:waveform(dbl)[], "AO Waveform (s)"=w337:waveform(dbl)[])
            n118 = local read "Channels"() -> (w339:T1[])
            n119 = for {
              tunnel: w342 -> [w365] mode=indexing
              tunnel: w340 -> [w364]
              shift-right: [w349] -> w335
              shift-left: w341 -> [w360]
              tunnel: [w348] -> w336
              i -> [w357]
              n120 = call-poly <vilib>:"Waveform to XY.vi"("error in (no error)"=w364, "Waveform in"=w365) -> ("error out"=w366:errorcluster, "XY-data out"=w367:cluster{"X-array":dbl[], "Y-array":dbl[]})  [unwired: 8 in]
              n121 = Increment(x=w357) -> (x+1=w359:i32)
              n122 = call-poly <vilib>:"Get X and Y.vi"("error in (no error)"=w366, "XY-data"=w367) -> ("error out"=w351:errorcluster, "Y-array"=w352:dbl[], "X-array"=w353:dbl[])  [unwired: 6 in, 1 out]
              n123 = Format Into String(format string="Ch%d" ("wavenames"), w359) -> (resulting string=w356:string)  [unwired: 2 in, 1 out]
              n124 = Concatenate Strings(w356, "_x" ("string")) -> (w362:string)
              n125 = call "Write Dictionary Element.vi"("error in (no error)"=w351, "value"=w353, "key"=w362, "Control Experiment in"=w360) -> ("error out"=w350:errorcluster, "Control Experiment out"=w361:refnum<class "Control Experiment.lvclass">)  [unwired: 6 in]
              n126 = Concatenate Strings(w356, "_y" ("string")) -> (w363:string)
              n127 = call "Write Dictionary Element.vi"("error in (no error)"=w350, "value"=w352, "key"=w363, "Control Experiment in"=w361) -> ("error out"=w348:errorcluster, "Control Experiment out"=w349:refnum<class "Control Experiment.lvclass">)  [unwired: 6 in]
            }
            n128 = Index Array(array=w339) -> (element=w333:T1)  [unwired: 1 in]
            n129 = Unbundle By Name(w333) -> ("Channel"=w326:u16)
            n130 = Decrement(x=w326) -> (x-1=w338:u16)
            n131 = Format Into String(format string="Sweep %d" ("wavenames"), w326) -> (resulting string=w331:string)  [unwired: 2 in, 1 out]
            n132 = Index Array(array=w337, index=w338) -> (element=w330:waveform(dbl))
            n133 = Unbundle By Name(w330) -> ("Y"=w329:dbl[])
            n134 = call "Write Dictionary Element.vi"("error in (no error)"=w336, "value"=w329, "key"=w331, "Control Experiment in"=w335) -> ("error out"=w334:errorcluster, "Control Experiment out"=w328:refnum<class "Control Experiment.lvclass">)  [unwired: 6 in]
            n135 = call "Exec State to Append.vi"("Execution:State"=w327) -> ("append?"=w325:bool)  [unwired: 2 in]
            n136 = call "Save Transport TDMS File.vi"("append?"=w325, "error in (no error)"=w334, "Control Experiment in"=w328) -> ("error out"=w343:errorcluster)  [unwired: 7 in, 1 out]
            n137 = call <vilib>:"Clear Errors.vi"("error in (no error)"=w343) -> ("error out"=w344:errorcluster)  [unwired: 5 in, 1 out]
            n138 = call <vilib>:"Add State(s) to Queue__jki_lib_state_machine.vi"("State(s) in (\"\")"=w347) -> ("States Out"=w346:string)  [unwired: 14 in]
          }
          frame "---------- Sweep ----------" {
            # "Template Separator\n(You can make a copy of, or modify, this frame)"
            n139 = call <vilib>:"Add State(s) to Queue__jki_lib_state_machine.vi"("State(s) in (\"\")"=w371) -> ("States Out"=w370:string)  [unwired: 14 in]
          }
          frame "Sweep: Initialize" {
            # "Template Separator\n(You can make a copy of, or modify, this frame)"
            n140 = Unbundle By Name(w376) -> ("Lockin"=w372)
            n141 = Bundle By Name(cluster=T7 {"Sweep Time (s)"=0.0, "Initial Wait (s)"=0.0, "Return to Start"=FALSE, "Channels"=[]} ("Configure Sweep"), "Sweep Time (s)"="Sweep Time (s)", "Initial Wait (s)"="Initial Wait (s)", "Return to Start"="Return to Start", "Channels"="Channels") -> (w382:T7)
            n142 = To More Specific Class(target class=refnum<class "Instrument.Lockin.lvclass"> refnum ("Instrument.Lockin in"), reference=w372) -> (specific class reference=w373:refnum<class "Instrument.Lockin.lvclass">)  [unwired: 1 in, 1 out]
            n143 = call-dynamic "setSweep.vi"("error in (no error)"=w385, "Configure Sweep"=w382, "Instrument.Lockin in"=w373) -> ("error out"=w384:errorcluster, "Instrument.Lockin out"=w377:refnum<class "Instrument.Lockin.lvclass">)  [unwired: 7 in]
            n144 = Bundle By Name(cluster=w376, "Lockin"=w377) -> (w375:T9)
            n145 = call <vilib>:"Add State(s) to Queue__jki_lib_state_machine.vi"("State(s) in (\"\")"=w387) -> ("States Out"=w386:string)  [unwired: 14 in]
          }
          frame "Sweep: Start" {
            # "wait for sweeping to start"
            # "Template Separator\n(You can make a copy of, or modify, this frame)"
            n146 = Unbundle By Name(w390) -> ("Lockin"=w395)
            n147 = call-dynamic "startSweep.vi"("error in (no error)"=w394, "Instrument.LockinAPI in"=w395) -> ("error out"=w392:errorcluster, "Instrument.LockinAPI out"=w393:refnum<class "Instrument.LockinAPI.lvclass">)  [unwired: 8 in]
            n148 = call-dynamic "waitStatusSweepingStarted.vi"("error in (no error)"=w392, "Instrument.LockinAPI in"=w393) -> ("error out"=w388:errorcluster, "Instrument.LockinAPI out"=w389:refnum<class "Instrument.LockinAPI.lvclass">)  [unwired: 8 in]
            n149 = Bundle By Name(cluster=w390, "Lockin"=w389) -> (w391:T9)
            n150 = call <vilib>:"Add State(s) to Queue__jki_lib_state_machine.vi"("State(s) in (\"\")"=w397) -> ("States Out"=w396:string)  [unwired: 14 in]
          }
          frame "Sweep: Stop" {
            # "Template Separator\n(You can make a copy of, or modify, this frame)"
            n151 = Unbundle By Name(w398) -> ("Lockin"=w403)
            n152 = call-dynamic "stopSweep.vi"("error in (no error)"=w402, "Instrument.LockinAPI in"=w403) -> ("error out"=w401:errorcluster, "Instrument.LockinAPI out"=w400:refnum<class "Instrument.LockinAPI.lvclass">)  [unwired: 8 in]
            n153 = Bundle By Name(cluster=w398, "Lockin"=w400) -> (w399:T9)
            n154 = call <vilib>:"Add State(s) to Queue__jki_lib_state_machine.vi"("State(s) in (\"\")"=w405) -> ("States Out"=w404:string)  [unwired: 14 in]
          }
          frame "Sweep: Check State" {
            # "Template Separator\n(You can make a copy of, or modify, this frame)"
            n155 = Unbundle By Name(w406) -> ("Lockin"=w412)
            n156 = call-dynamic "getStatus.vi"("error in (no error)"=w411, "Instrument.LockinAPI in"=w412) -> ("error out"=w410:errorcluster, "state"=w413:T12, "Instrument.LockinAPI out"=w408:refnum<class "Instrument.LockinAPI.lvclass">)  [unwired: 7 in]
            "Status" <- w413
            n157 = case shown="\"sweeping\"" w413 {
              tunnel: ["Macro: Exit" ("State(s) in Front (\"\")") "Macro: Sweep" ("State(s) in Front (\"\")")] -> w409
              frame Default {
              }
              frame "sweeping" {
              }
            }
            n158 = Bundle By Name(cluster=w406, "Lockin"=w408) -> (w407:T9)
            n159 = call <vilib>:"Add State(s) to Queue__jki_lib_state_machine.vi"("State(s) in Front (\"\")"=w409, "State(s) in (\"\")"=w415) -> ("States Out"=w414:string)  [unwired: 13 in]
          }
          frame "---------- Measure ----------" {
            # "Do not put any code in this frame.\n(It is a separator no-op. You can make a copy of this frame to create a new Macro frame)"
            n160 = call <vilib>:"Add State(s) to Queue__jki_lib_state_machine.vi"("State(s) in (\"\")"=w421) -> ("States Out"=w420:string)  [unwired: 14 in]
          }
          frame "Measure: Time" {
            # "Do not put any code in this frame.\n(It is a separator no-op. You can make a copy of this frame to create a new Macro frame)"
            n161 = Unbundle By Name(w428) -> ("C.E."=w427:refnum<class "Control Experiment.lvclass">)
            n162 = Get Date/Time In Seconds() -> (seconds since 1Jan1904=w430:timestamp)
            n163 = To Double Precision Float(number=w430) -> (double precision float=w423:dbl)
            n164 = call "Append Dictionary Element.vi"("error in (no error)"=w425, "value"=w423, "key"="Time", "Control Experiment in"=w427) -> ("error out"=w422:errorcluster, "Control Experiment out"=w426:refnum<class "Control Experiment.lvclass">)  [unwired: 6 in]
            n165 = Bundle By Name(cluster=w428, "C.E."=w426) -> (w429:T9)
            n166 = call <vilib>:"Add State(s) to Queue__jki_lib_state_machine.vi"("State(s) in (\"\")"=w432) -> ("States Out"=w431:string)  [unwired: 14 in]
          }
          frame "Measure: Temperature" {
            # "Do not put any code in this frame.\n(It is a separator no-op. You can make a copy of this frame to create a new Macro frame)"
            n167 = Unbundle By Name(w441) -> ("C.E."=w436:refnum<class "Control Experiment.lvclass">, "Instruments.Temperature"=w443:refnum<class "Instrument.Cryostat.lvclass">)
            n168 = call-dynamic "Get Temperature.vi"("error in (no error)"=w442, "Instrument.Cryostat in"=w443) -> ("error out"=w437:errorcluster, "Temperature (K)"=w438:dbl, "Instrument.Cryostat out"=w433:refnum<class "Instrument.Cryostat.lvclass">)  [unwired: 5 in, 2 out]
            n169 = call "Append Dictionary Element.vi"("error in (no error)"=w437, "value"=w438, "key"="Temperature", "Control Experiment in"=w436) -> ("error out"=w434:errorcluster, "Control Experiment out"=w435:refnum<class "Control Experiment.lvclass">)  [unwired: 6 in]
            n170 = Bundle By Name(cluster=w441, "Instruments.Temperature"=w433, "C.E."=w435) -> (w440:T9)
            n171 = call <vilib>:"Add State(s) to Queue__jki_lib_state_machine.vi"("State(s) in (\"\")"=w445) -> ("States Out"=w444:string)  [unwired: 14 in]
          }
          frame "Measure: Magnet" {
            # "Do not put any code in this frame.\n(It is a separator no-op. You can make a copy of this frame to create a new Macro frame)"
            n172 = Unbundle By Name(w456) -> ("C.E."=w453:refnum<class "Control Experiment.lvclass">, "Instruments.Temperature"=w448:refnum<class "Instrument.Cryostat.lvclass">)
            n173 = call-dynamic "Get Magnet.vi"("error in (no error)"=w450, "Instrument.Cryostat in"=w448) -> ("error out"=w449:errorcluster, "B Field (T)"=w447:dbl, "Instrument.Cryostat out"=w446:refnum<class "Instrument.Cryostat.lvclass">)  [unwired: 5 in, 2 out]
            n174 = call "Append Dictionary Element.vi"("error in (no error)"=w449, "value"=w447, "key"="Magnet", "Control Experiment in"=w453) -> ("error out"=w451:errorcluster, "Control Experiment out"=w452:refnum<class "Control Experiment.lvclass">)  [unwired: 6 in]
            n175 = Bundle By Name(cluster=w456, "Instruments.Magnet"=w446, "C.E."=w452) -> (w455:T9)
            n176 = call <vilib>:"Add State(s) to Queue__jki_lib_state_machine.vi"("State(s) in (\"\")"=w458) -> ("States Out"=w457:string)  [unwired: 14 in]
          }
          frame "Measure: Lockin" {
            # "Do not put any code in this frame.\n(It is a separator no-op. You can make a copy of this frame to create a new Macro frame)"
            n177 = Unbundle By Name(w470) -> ("t0"=w467:timestamp, "AI Waveform (s)"=w463:waveform(dbl)[], "Lockin"=w466, "AO Waveform (s)"=w460:waveform(dbl)[])
            n178 = Array Size(array=w463) -> (size(s)=w462:i32)
            n179 = case shown="0" w462 {
              tunnel: w463 -> [_ w505]
              tunnel: [w479 w504] -> w469
              tunnel: [w474 w503] -> w464
              tunnel: w465 -> [w483 w502]
              tunnel: [w480 w499] -> w468
              tunnel: w466 -> [w484 w498]
              tunnel: w467 -> [_ w496]
              tunnel: [w476 w492] -> w461
              tunnel: w460 -> [_ w493]
              tunnel: [w475 w491] -> w459
              frame 0 {
                n180 = for {
                  N: 3 -> [_]
                  tunnel: [w487] -> w479
                  tunnel: w483 -> [w488]
                  tunnel: [w486] -> w478
                  shift-right: [w485] -> w477
                  shift-left: w484 -> [w489]
                  n181 = call-dynamic "waitNewWaveforms.vi"("error in (no error)"=w488, "Instrument.LockinAPI in"=w489) -> ("error out"=w486:errorcluster, "Newest AI Waveform"=w487:waveform(dbl)[], "Instrument.LockinAPI out"=w485:refnum<class "Instrument.LockinAPI.lvclass">)  [unwired: 7 in]
                }
                n182 = call-dynamic "getAOwfm.vi"("error in (no error)"=w478, "Instrument.LockinAPI in"=w477) -> ("error out"=w474:errorcluster, "AO Waveforrm"=w476:waveform(dbl)[], "Instrument.LockinAPI out"=w475:refnum<class "Instrument.LockinAPI.lvclass">)  [unwired: 7 in]
                n183 = Index Array(array=w479) -> (element=w482:waveform(dbl))  [unwired: 1 in]
                n184 = Unbundle By Name(w482) -> ("t0"=w480:timestamp)
              }
              frame Default {
                n185 = call-dynamic "getAIwfm.vi"("error in (no error)"=w502, "Instrument.LockinAPI in"=w498) -> ("error out"=w490:errorcluster, "AI Waveform"=w497:waveform(dbl)[], "Instrument.LockinAPI out"=w495:refnum<class "Instrument.LockinAPI.lvclass">)  [unwired: 7 in]
                n186 = Index Array(array=w497) -> (element=w501:waveform(dbl))  [unwired: 1 in]
                n187 = call-dynamic "getAOwfm.vi"("error in (no error)"=w490, "Instrument.LockinAPI in"=w495) -> ("AO Waveforrm"=w494:waveform(dbl)[], "Instrument.LockinAPI out"=w491:refnum<class "Instrument.LockinAPI.lvclass">)  [unwired: 7 in, 1 out]
                n188 = Unbundle By Name(w501) -> ("t0"=w499:timestamp)
                n189 = Equal?(x=w499, y=w496) -> (x = y?=w500:bool)
                n190 = case shown="False" w500 {
                  tunnel: w505 -> [w510 w537]
                  tunnel: [w513 w537] -> w504
                  tunnel: [w512 w538] -> w503
                  tunnel: w490 -> [w511 w538]
                  tunnel: w497 -> [w514 _]
                  tunnel: w494 -> [w508 _]
                  tunnel: w493 -> [w507 w536]
                  tunnel: [w506 w536] -> w492
                  frame False {
                    n191 = Array Size(array=w510) -> (size(s)=w509:i32)
                    n192 = case shown="Default" w509 {
                      tunnel: w514 -> [w517 w525]
                      tunnel: [w517 w524] -> w513
                      tunnel: [w516 w523] -> w512
                      tunnel: w511 -> [w516 w519]
                      tunnel: w510 -> [_ w522]
                      tunnel: w508 -> [_ w521]
                      tunnel: w507 -> [w515 w520]
                      tunnel: [w515 w518] -> w506
                      frame 0 {
                      }
                      frame Default {
                        n193 = for {
                          tunnel: w522 -> [w531] mode=indexing
                          tunnel: w525 -> [w535] mode=indexing
                          tunnel: [w534] -> w524 mode=indexing
                          tunnel: [w533] -> w523
                          tunnel: w519 -> [w532]
                          n194 = call-poly <vilib>:"Append Waveforms.vi"("error in (no error)"=w532, "waveform B"=w535, "waveform A"=w531) -> ("error out"=w533:errorcluster, "waveform out"=w534:waveform(dbl))  [unwired: 7 in]
                        }
                        n195 = for {
                          tunnel: w520 -> [w526] mode=indexing
                          tunnel: w521 -> [w530] mode=indexing
                          tunnel: [w529] -> w518 mode=indexing
                          tunnel: [w528] -> _
                          tunnel: w519 -> [w527]
                          n196 = call-poly <vilib>:"Append Waveforms.vi"("error in (no error)"=w527, "waveform B"=w530, "waveform A"=w526) -> ("error out"=w528:errorcluster, "waveform out"=w529:waveform(dbl))  [unwired: 7 in]
                        }
                      }
                    }
                  }
                  frame True {
                  }
                }
              }
            }
            n197 = Bundle By Name(cluster=w470, "t0"=w468, "AI Waveform (s)"=w469, "AO Waveform (s)"=w461, "Lockin"=w459) -> (w471:T9)
            n198 = call <vilib>:"Add State(s) to Queue__jki_lib_state_machine.vi"("State(s) in (\"\")"=w473) -> ("States Out"=w472:string)  [unwired: 14 in]
          }
        }
      }
      "error out" <- w3
      n199 = Unbundle By Name(w2) -> ("Transport"=→"Transport.lvclass":refnum<class "Transport.lvclass">)
    }
    frame Enabled {
    }
  }
